vi "Update Info.vi"(7 "State":T1, 8 "error in (no error)":errorcluster, 9 "Col":i32, 10 "Row":i32, 11 "2DPanelBlank in":refnum<class "2DPanelBlank.lvclass">) -> (0 "error out":errorcluster, 3 "2DPanelBlank out":refnum<class "2DPanelBlank.lvclass">)   [LabVIEW 2020, in "OOPanel.lvlib" / "2DPanelBlank.lvclass"]
uses:
  2DPanelBlank.lvclass
  State.ctl
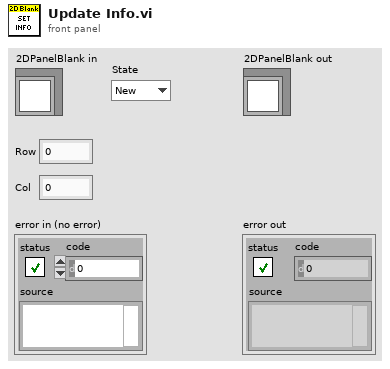
[diagram p1: front panel]
types:
  T1 = typedef "OOPanel.lvlib/2DPanelBlank.lvclass/State.ctl" = enum16{"New", "Idle", "Pool", "Used", "No SP"}
  T2 = typedef "OOPanel.lvlib/2DPanelBlank.lvclass/Info.ctl" = cluster{"Index":T3, "State":T1, "Pull Count":i32}
  T3 = typedef "OOPanel.lvlib/2D Index.ctl" = cluster{"Row":i32, "Col":i32}
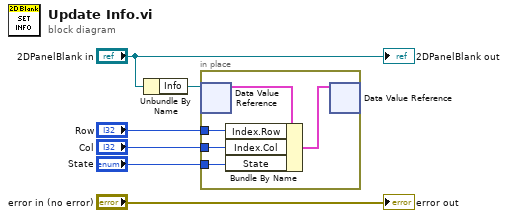
[diagram p0: block diagram]
diagram:
  n1 = Unbundle By Name("2DPanelBlank in") -> ("Info"=w5:refnum<data-value>)
  n2 = in-place {
    in-place-border: "Row" -> [w9]
    in-place-border: "Col" -> [w8]
    in-place-border: "State" -> [w7]
    n3 = in-place-dvr #1(w5) -> (w11:T2)  [unwired: 1 out]
    n4 = Bundle By Name(cluster=w11, "Index.Row"=w9, "Index.Col"=w8, "State"=w7) -> (w10:T2)
    n5 = in-place-dvr #1(w10) -> ()  [unwired: 2 out]
  }
  "error out" <- "error in (no error)"
  "2DPanelBlank out" <- "2DPanelBlank in"
